vi "ExampleAutoMessageFGV.vi"() -> ()   [LabVIEW 2019, in "MicronTemplateCore.lvclass"]
doc: "This is the VI description for the Add command, which can be queried by a client with\nCommand : Help, Payload: Add."
uses:
  MicronTemplateCore.lvclass
panel:
  out "Numeric3":dbl
  in  "Numeric2":dbl
  in  "Numeric1":dbl
  # "Multiply Two Numbers"
  # "The name of the VI, the list of controls names and data types in this server side API should exactly match the control names on the client side API.\n\nRefer to MicronTemplateAPIs\\Examples\\ExampleAutoMessageFGV.vi"
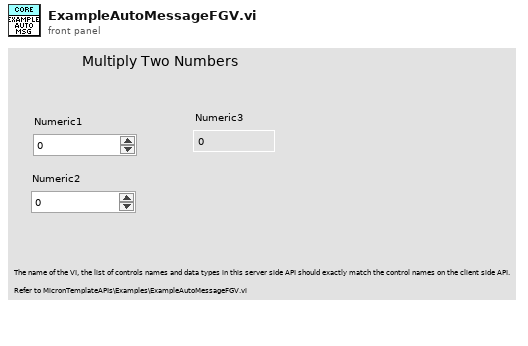
[diagram p1: front panel]
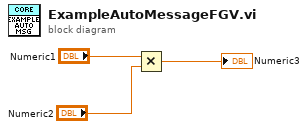
[diagram p0: block diagram]
diagram:
  n1 = Multiply(x="Numeric1", y="Numeric2") -> (x*y=→"Numeric3":dbl)
